vi "subLLSE.vi"(0 "A":cdb[][](array[numeric])=[[1.0+0.0i, 0.0+0.0i, 0.0+0.0i], [0.0+0.0i, 1.0+0.0i, 0.0+0.0i], [0.0+0.0i, 0.0+0.0i, 1.0+0.0i], [0.0+0.0i, 0.0+0.0i, 0.0+0.0i], [0.0+0.0i, 0.0+0.0i, 0.0+0.0i]], 5 "b":cdb[](array[numeric])=[1.0+0.0i, 1.0+0.0i, 1.0+0.0i, 0.0+0.0i, 0.0+0.0i], 11 "error in (no error)":errorcluster) -> (4 "x.estimate":cdb[](array[numeric]), 6 "mean square error":dbl, 15 "error out":errorcluster)   [LabVIEW 2011]
uses:
  <vilib>/Analysis/_algsub.llb/Complex Vector Norm.vi
  <vilib>/Analysis/baseanly.llb/Complex A x Vector.vi
  <vilib>/Analysis/baseanly.llb/Complex A x B.vi
  <vilib>/Analysis/baseanly.llb/Complex Inverse Matrix.vi
  <vilib>/Analysis/7linalg.llb/Complex Conjugate Transpose Matrix.vi
  <vilib>/Analysis/NI_AALPro.lvlib
  <vilib>/Analysis/NI_AALBase.lvlib
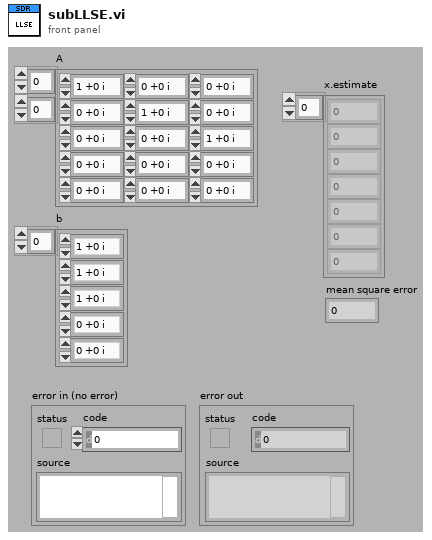
[diagram p1: front panel]
types:
  T1 = typedef "NI_Matrix.lvlib/ComplexMatrix.ctl" = cdb[][]
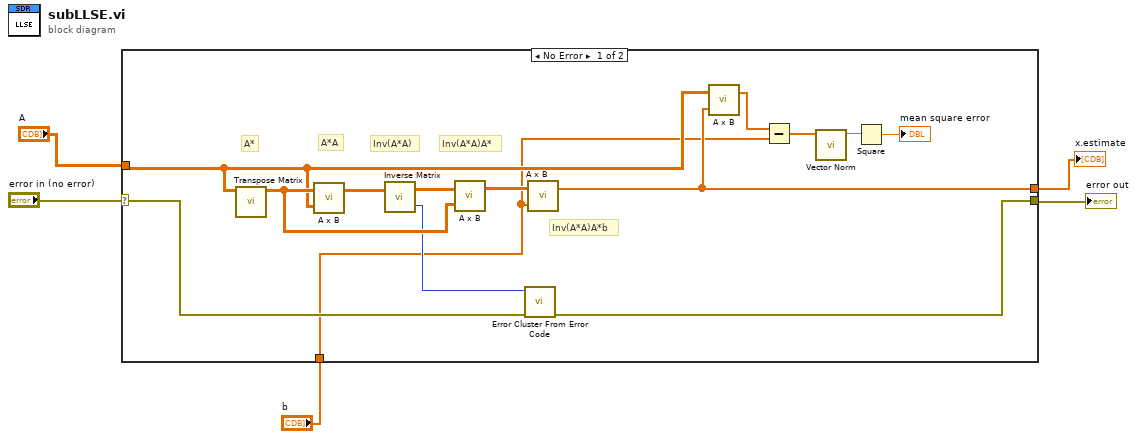
[diagram p0: block diagram]
diagram:
  n1 = case shown="No Error" "error in (no error)" {
    selector: "error in (no error)" -> [w11 w20]
    tunnel: [w9 w20] -> w4
    tunnel: "A" -> [w8 _]
    tunnel: [w7 _] -> w2
    tunnel: "b" -> [w6 _]
    frame No Error {
      # "Inv(A*A)A*b"
      # "Inv(A*A)A*"
      # "Inv(A*A)"
      # "A*A"
      # "A*"
      n2 = call-poly <vilib>:"Transpose Matrix.vi"("Input Matrix"=w8) -> ("Matrix Conjugate Transpose"=w17:T1)  [unwired: 10 out]
      n3 = call-poly <vilib>:"A x B.vi"("B"=w8, "A"=w17) -> ("A x B"=w19:T1)  [unwired: 1 out]
      n4 = call-poly <vilib>:"Inverse Matrix.vi"("Input Matrix"=w19) -> ("error"=w10:i32, "Inverse Matrix"=w18:T1)  [unwired: 1 in]
      n5 = call-poly <vilib>:"A x B.vi"("B"=w17, "A"=w18) -> ("A x B"=w16:T1)  [unwired: 1 out]
      n6 = call <vilib>:"Error Cluster From Error Code.vi"("error in (no error)"=w11, "error code (0)"=w10) -> ("error out"=w9:errorcluster)  [unwired: 7 in]
      n7 = call-poly <vilib>:"A x B.vi"("Vector"=w6, "A"=w16) -> ("A x Vector"=w7:cdb[])  [unwired: 1 out]
      n8 = call-poly <vilib>:"A x B.vi"("Vector"=w7, "A"=w8) -> ("A x Vector"=w15:cdb[])  [unwired: 1 out]
      n9 = Subtract ("Subtract.vi")(x=w15, y=w6) -> (x-y=w14:cdb[])
      n10 = call-poly <vilib>:"Vector Norm.vi"("Input Vector"=w14) -> ("norm"=w13:dbl)  [unwired: 2 in, 8 out]
      n11 = Square(x=w13) -> (x^2=→"mean square error":dbl)
    }
    frame Error {
    }
  }
  "error out" <- w4
  "x.estimate" <- w2
